vi "Alessi.vi"() -> ()   [LabVIEW 2018, in "AlessiRel6100.lvclass"]
uses:
  AlessiRel6100.lvclass
panel:
  out "Alessi Probestation Configurations":T1={"Device ID Probe Station"=2, "Ref No."=0, "Touchdown method"=enum."no feedback", "Arduino Edgesense params"={"touchdown height [µm]"=0, "search band [µm]"=100, "speed [µm/step]"=10, "overdrive [µm]"=30}}
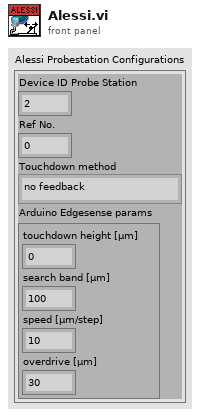
[diagram p1: front panel]
types:
  T1 = cluster{"Device ID Probe Station":u32, "Ref No.":u32, "Touchdown method":enum16{"no feedback", "Arduino edgesense"}, "Arduino Edgesense params":cluster{"touchdown height [µm]":i32, "search band [µm]":u32, "speed [µm/step]":u32, "overdrive [µm]":u32}}
diagram:
